vi "Configuration UI.vi"(8 "error in (no error)":errorcluster, 11 "Base Step in":refnum<class "Base Step.lvclass">) -> (0 "error out":errorcluster, 2 "JSON Configuration":string, 3 "Base Step out":refnum<class "Base Step.lvclass">)   [LabVIEW 2024, in "Ramses Sequencer.lvlib" / "Base Step.lvclass"]
uses:
  Base Step.lvclass
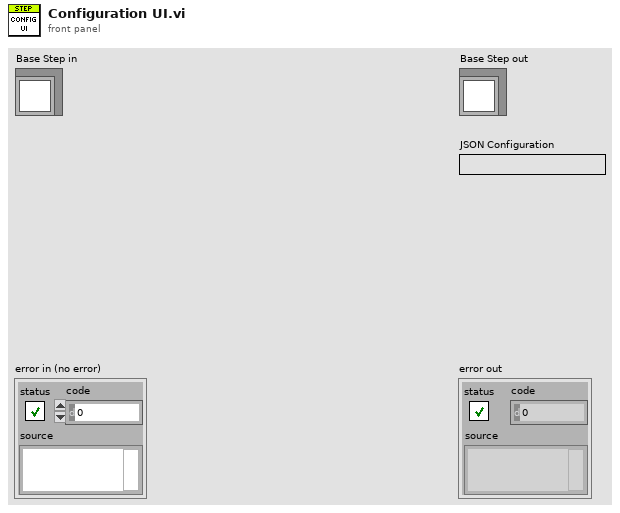
[diagram p1: front panel]
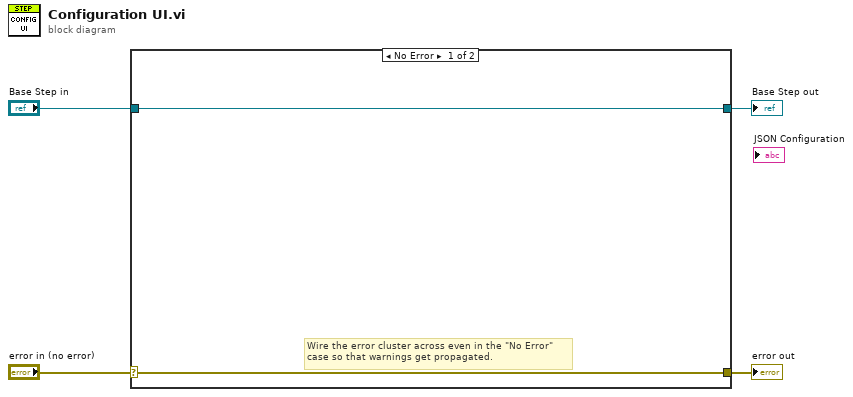
[diagram p0: block diagram]
diagram:
  n1 = case shown="No Error" "error in (no error)" {
    selector: "error in (no error)" -> [w5 w8]
    tunnel: [w5 w8] -> w3
    tunnel: [w6 w7] -> w1
    tunnel: "Base Step in" -> [w6 w7]
    frame No Error {
      # "Wire the error cluster across even in the \"No Error\"\ncase so that warnings get propagated."
    }
    frame Error {
    }
  }
  "error out" <- w3
  "Base Step out" <- w1
